vi "smoothing_algo.vi"() -> ()   [LabVIEW 2012]
uses:
  <vilib>/Analysis/6fits.llb/Curve Fitting Criteria.ctl
  <vilib>/Analysis/6fits.llb/General Linear Fit Algorithm.ctl
  <vilib>/Analysis/NI_AALPro.lvlib
panel:
  out "Polynomial Coefficients":dbl[](array[numeric])
  in  "polynomial order":i32=2
  in  "algorithm":T1 items=["SVD", "Givens", "Givens2", "Householder", "LU Decomposition", "Cholesky", "SVD for Rank Deficient H"]
  in  "method":T2 items=["Least Square", "Least Absolute Residual", "Bisquare"]
  in  "parameter selection":u16(ring)=2 items=["equally spaced", "chord length", "centripetal"]
  in  "degree":i32=3
  in  "# of control points":i32=10
  out "XY Graph":cluster{dbl[], dbl[]}[](graph)
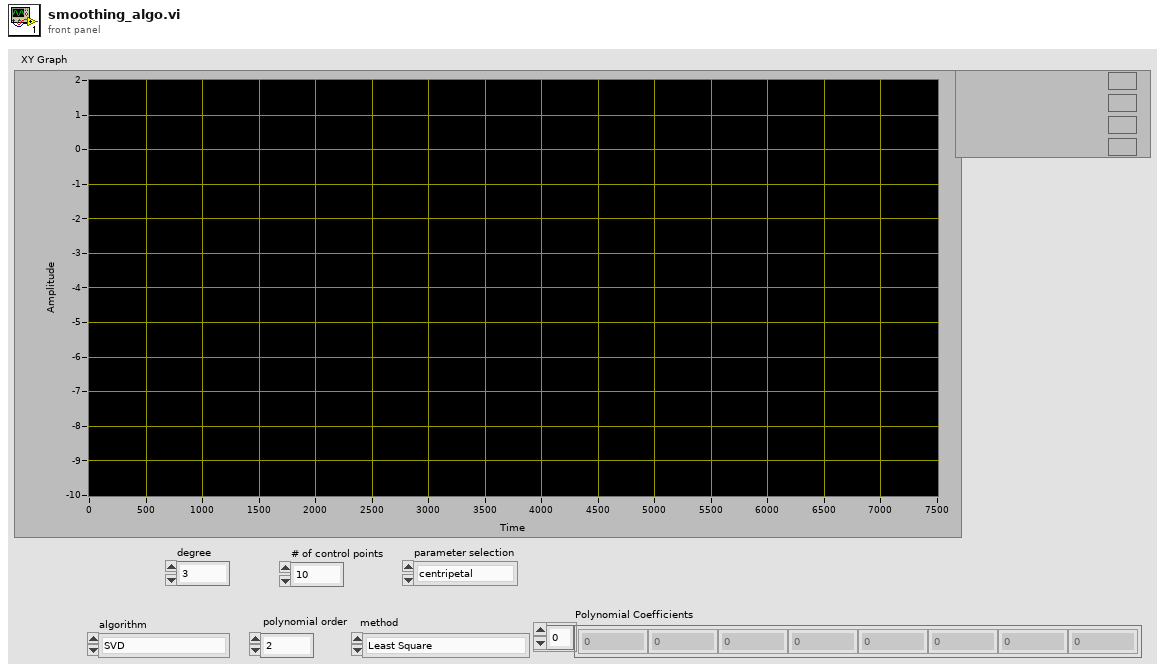
[diagram p1: front panel]
types:
  T1 = typedef "NI_AALPro.lvlib/General Linear Fit Algorithm.ctl" = u16
  T2 = typedef "NI_AALPro.lvlib/Curve Fitting Criteria.ctl" = u16
  T3 = cluster{"Best BSpline Fit X":dbl[], "Best BSpline Fit Y":dbl[]}
  T4 = cluster{"Best BSpline Fit X":dbl[], "Best Polynomial Fit":dbl[]}[]
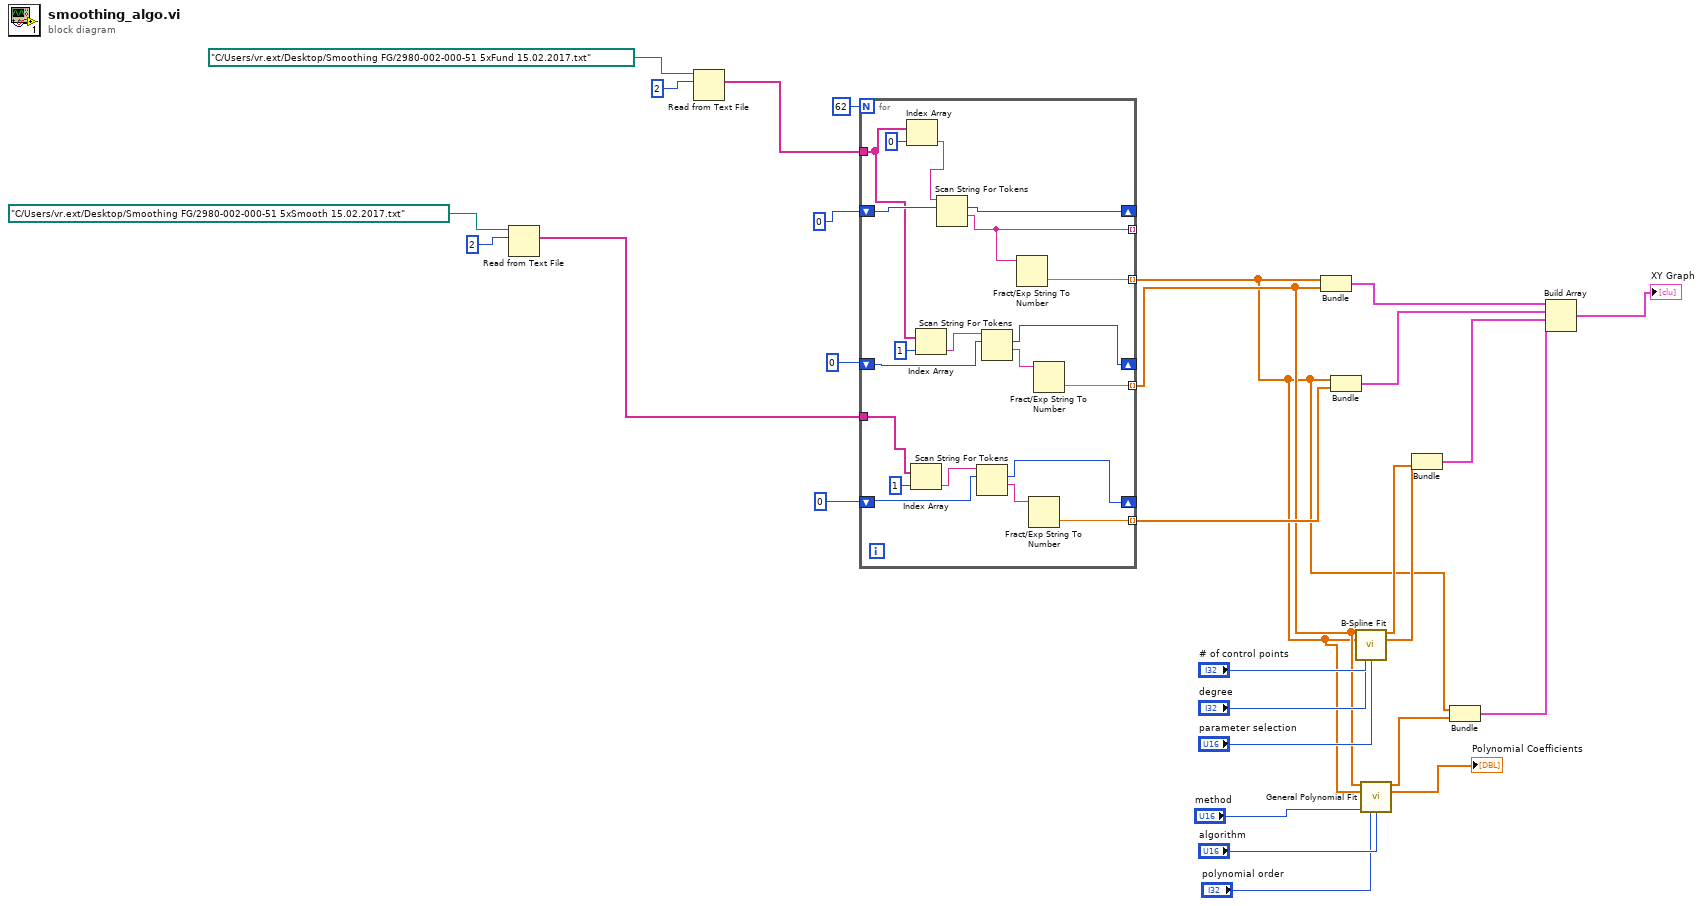
[diagram p0: block diagram]
diagram:
  n1 = Read from Text File(file (use dialog)=path "C:/Users/vr.ext/Desktop/Smoothing FG/2980-002-000-51 5xSmooth 15.02.2017.txt", count=2) -> (text=w20:string[])  [unwired: 2 in, 3 out]
  n2 = Read from Text File(file (use dialog)=path "C:/Users/vr.ext/Desktop/Smoothing FG/2980-002-000-51 5xFund 15.02.2017.txt", count=2) -> (text=w26:string[])  [unwired: 2 in, 3 out]
  n3 = for {
    N: 62 -> [_]
    tunnel: w26 -> [w41]
    shift-right: [w47] -> _
    shift-left: 0 ("count") -> [w48]
    tunnel: [w44] -> _ mode=indexing
    tunnel: [w43] -> w6 mode=indexing
    shift-right: [w38] -> _
    shift-left: 0 ("count") -> [w39]
    tunnel: [w36] -> w8 mode=indexing
    tunnel: w20 -> [w32]
    shift-right: [w30] -> _
    shift-left: 0 ("count") -> [w31]
    tunnel: [w29] -> w18 mode=indexing
    n4 = Index Array(array=w41, index=0) -> (element=w46:string)
    n5 = Index Array(array=w32, index=1) -> (element=w34:string)
    n6 = Index Array(array=w41, index=1) -> (element=w40:string)
    n7 = Scan String For Tokens(8:w48, 9:w46) -> (1:w44:string, 2:w47:i32)  [unwired: 4 in, 2 out]
    n8 = Scan String For Tokens(8:w31, 9:w34) -> (1:w35:string, 2:w30:i32)  [unwired: 4 in, 2 out]
    n9 = Scan String For Tokens(8:w39, 9:w40) -> (1:w37:string, 2:w38:i32)  [unwired: 4 in, 2 out]
    n10 = Fract/Exp String To Number(string=w44) -> (number=w43:dbl)  [unwired: 3 in, 1 out]
    n11 = Fract/Exp String To Number(string=w35) -> (number=w29:dbl)  [unwired: 3 in, 1 out]
    n12 = Fract/Exp String To Number(string=w37) -> (number=w36:dbl)  [unwired: 3 in, 1 out]
  }
  n13 = Bundle(w6, w8) -> (w17:cluster{dbl[], dbl[]})  [unwired: 1 in]
  n14 = Bundle(w6, w18) -> (w16:cluster{dbl[], dbl[]})  [unwired: 1 in]
  n15 = call <vilib>:"B-Spline Fit.vi"("Y"=w8, "# of control points"="# of control points", "X"=w6, "degree"="degree", "parameter selection"="parameter selection") -> ("Best BSpline Fit Y"=w11:dbl[], "Best BSpline Fit X"=w10:dbl[])  [unwired: 7 in, 2 out]
  n16 = call <vilib>:"General Polynomial Fit.vi"("Y"=w8, "polynomial order"="polynomial order", "X"=w6, "method"="method", "algorithm"="algorithm") -> ("Best Polynomial Fit"=w7:dbl[], "Polynomial Coefficients"=→"Polynomial Coefficients":dbl[])  [unwired: 7 in, 2 out]
  n17 = Bundle("Best BSpline Fit X"=w10, "Best BSpline Fit Y"=w11) -> (w9:T3)  [unwired: 1 in]
  n18 = Bundle(w6, "Best Polynomial Fit"=w7) -> (w5:cluster{dbl[], "Best Polynomial Fit":dbl[]})  [unwired: 1 in]
  n19 = Build Array(w17, w16, w9, w5) -> (→"XY Graph":T4)
